vi "SLSC Search and Convert ENUM Value by Name.vi"(6 "Enum Strings":cluster{"name":string, string}[](array[cluster]), 9 "enums":T1[](array[typedef]), 10 "Value":string, 11 "Datatype Name":string) -> (1 "Enum":T1, 2 "Datatype found?":bool, 3 "Value":i32)   [LabVIEW 2020, in "SLSC Tree Control.lvlib"]
doc: "Search and convert a ENUM datatype based on the name of the item."
uses:
  SLSC Tree Control.lvlib
  SLSC EDS API/JSON parsing/enum.ctl
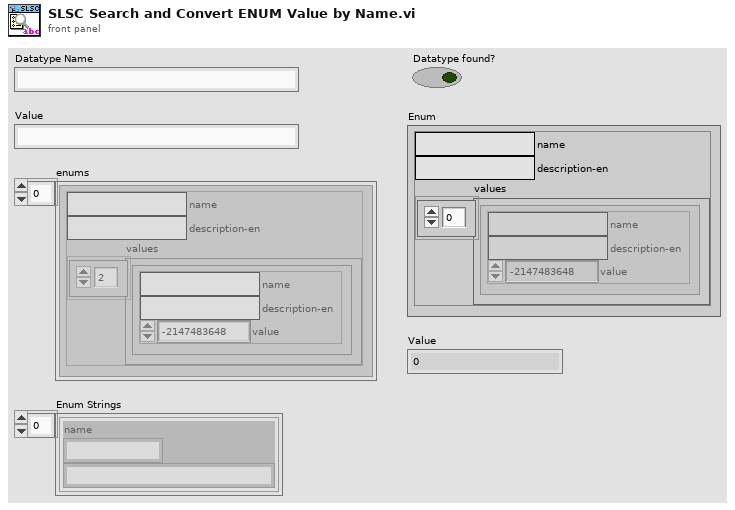
[diagram p1: front panel]
types:
  T1 = typedef "enum.ctl" = cluster{"name":string, "description-en":string, "values":cluster{"name":string, "description-en":string, "value":i32}[]}
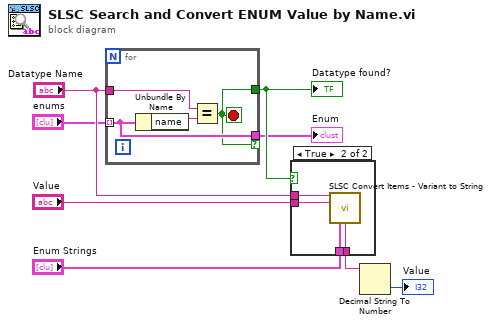
[diagram p0: block diagram]
diagram:
  n1 = for {
    tunnel: "enums" -> [w10] mode=indexing
    tunnel: "Datatype Name" -> [w11]
    tunnel: [w10] -> w2 if=w9
    tunnel: [w9] -> w4
    stop <- w9 stop-if-true
    n2 = Unbundle By Name(w10) -> ("name"=w12:string)
    n3 = Equal?(x=w11, y=w12) -> (x = y?=w9:bool)
  }
  "Datatype found?" <- w4
  "Enum" <- w2
  n4 = case shown="True" w4 {
    tunnel: "Value" -> [w13 w14]
    tunnel: [w13 w17] -> w5
    tunnel: "Enum Strings" -> [_ w16]
    tunnel: "Datatype Name" -> [_ w15]
    frame False {
    }
    frame True {
      n5 = call "SLSC Convert Items - Variant to String.vi"("Datatype"=w15, "value"=w14, "Enum string"=w16) -> ("Option"=w17:string)  [unwired: 6 in, 6 out]
    }
  }
  n6 = Decimal String To Number(string=w5) -> (number=→"Value":i32)  [unwired: 2 in, 1 out]
